vi "Modbus LDO Boolean Decode.vi"(8 "error in":errorcluster, 11 "PLC Data":T1) -> (0 "error out":errorcluster, 3 "PLC Data Out":T1)   [LabVIEW 2020, in "Modbus.lvlib"]
uses:
  Modbus.lvlib
  Modbus PLC Data All.ctl
  Modbus FVIR Control.ctl
  Modbus LDO Control.ctl
  WritingDataFile/Data to Save.ctl
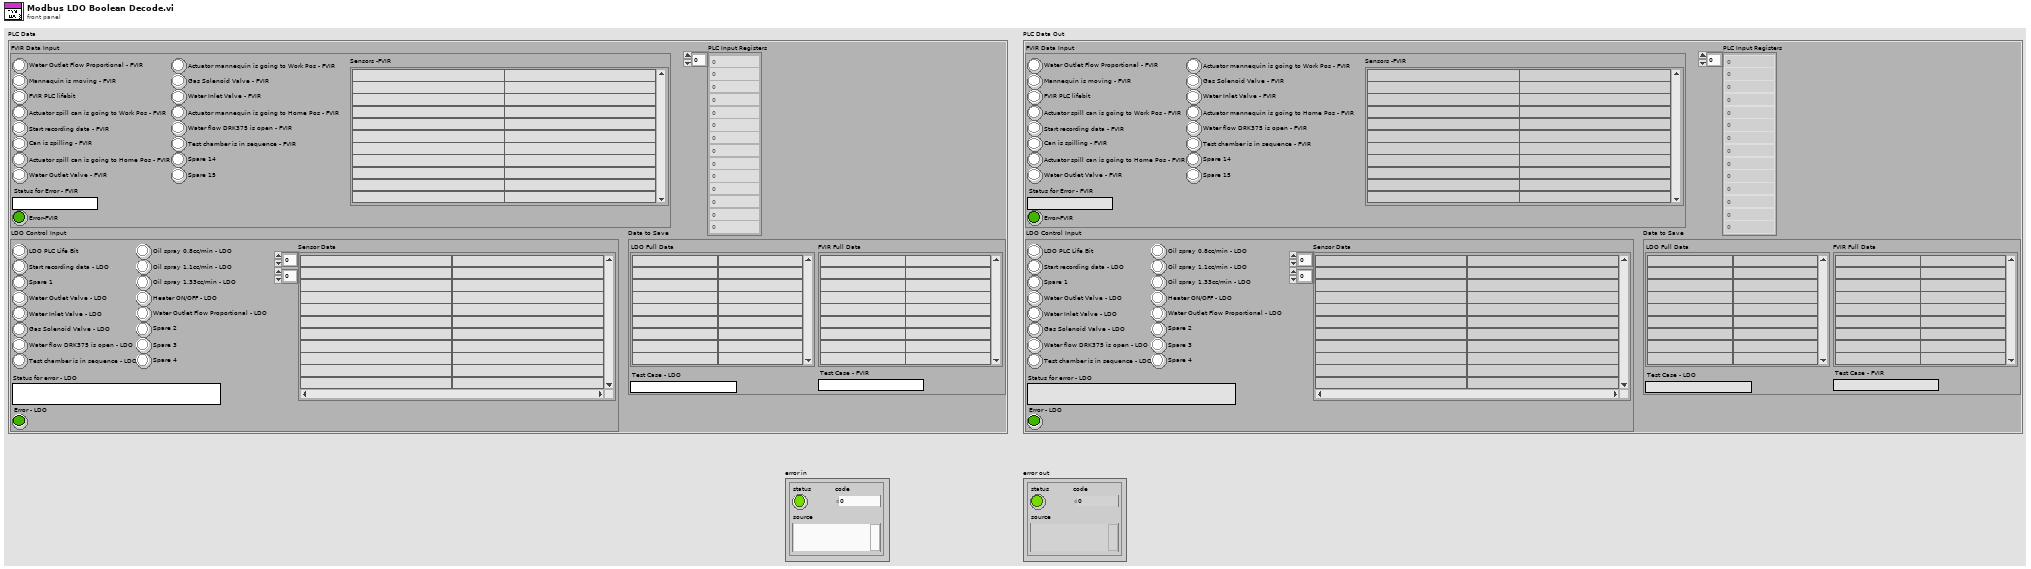
[diagram p1: front panel]
types:
  T1 = typedef "Modbus PLC Data All.ctl" = cluster{"FVIR Data Input":T2, "LDO Control Input":T3, "PLC Input Registers":u16[], "Data to Save":T4}
  T2 = typedef "Modbus FVIR Control.ctl" = cluster{"Spare 15":bool, "Spare 14":bool, "Actuator mannequin is going to Work Pos - FVIR":bool, "Actuator mannequin is going to Home Pos - FVIR":bool, "Test chamber is in sequence - FVIR ":bool, "Water flow DRK375 is open - FVIR":bool, "Gas Solenoid Valve - FVIR":bool, "Water Inlet Valve - FVIR":bool, "Water Outlet Flow Proportional - FVIR":bool, "Start recording data - FVIR":bool, "Actuator spill can is going to Work Pos - FVIR":bool, "Actuator spill can is going to Home Pos - FVIR":bool, "Water Outlet Valve - FVIR":bool, "Can is spilling - FVIR":bool, "Mannequin is moving - FVIR":bool, "FVIR PLC lifebit":bool, "Status for Error - FVIR":string, "Error-FVIR":bool, "Sensors -FVIR":string[][]}
  T3 = typedef "Modbus LDO Control.ctl" = cluster{"LDO PLC Life Bit":bool, "Start recording data - LDO":bool, "Spare 1":bool, "Water Outlet Valve - LDO":bool, "Water Inlet Valve - LDO":bool, "Gas Solenoid Valve - LDO":bool, "Water flow DRK375 is open - LDO":bool, "Test chamber is in sequence - LDO":bool, "Oil spray 0.8cc/min - LDO":bool, "Oil spray 1.1cc/min - LDO":bool, "Oil spray 1.33cc/min - LDO":bool, "Heater ON/OFF - LDO":bool, "Water Outlet Flow Proportional - LDO":bool, "Spare 2":bool, "Spare 3":bool, "Spare 4":bool, "Status for error - LDO":string, "Error - LDO":bool, "Sensor Data":string[][]}
  T4 = typedef "Data to Save.ctl" = cluster{"LDO Full Data":string[][], "FVIR Full Data":string[][], "Test Case - FVIR":string, "Test Case - LDO":string}
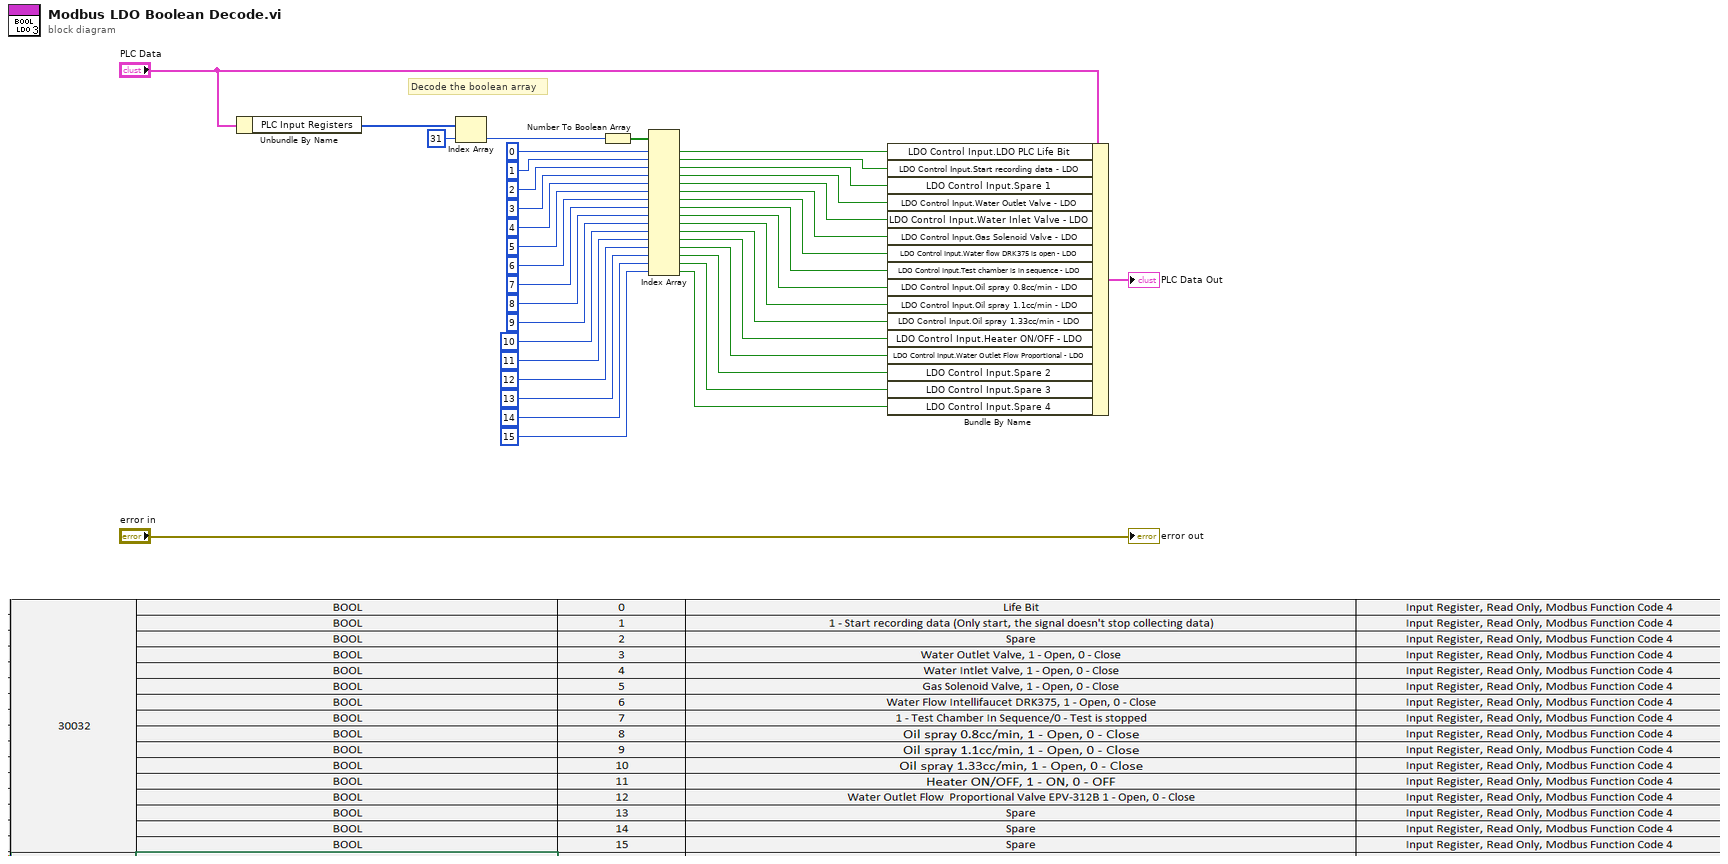
[diagram p0: block diagram]
diagram:
  # "Decode the boolean array"
  n1 = Unbundle By Name("PLC Data") -> ("PLC Input Registers"=w2:u16[])
  n2 = Index Array(array=w2, index=31) -> (element=w39:u16)
  n3 = Number To Boolean Array(number=w39) -> (Boolean array=w38:bool[])
  n4 = Index Array(array=w38, index #1=0 ("index"), index #2=1 ("index"), index #3=2 ("index"), index #4=3 ("index"), index #5=4 ("index"), index #6=5 ("index"), index #7=6 ("index"), index #8=7 ("index"), index #9=8 ("index"), index #10=9 ("index"), index #11=10 ("index"), index #12=11 ("index"), index #13=12 ("index"), index #14=13 ("index"), index #15=14 ("index"), index #16=15 ("index")) -> (element #1=w20:bool, element #2=w19:bool, element #3=w18:bool, element #4=w17:bool, element #5=w16:bool, element #6=w15:bool, element #7=w14:bool, element #8=w13:bool, element #9=w12:bool, element #10=w11:bool, element #11=w10:bool, element #12=w9:bool, element #13=w8:bool, element #14=w7:bool, element #15=w6:bool, element #16=w5:bool)
  n5 = Bundle By Name(cluster="PLC Data", "LDO Control Input.LDO PLC Life Bit"=w20, "LDO Control Input.Start recording data - LDO"=w19, "LDO Control Input.Spare 1"=w18, "LDO Control Input.Water Outlet Valve - LDO"=w17, "LDO Control Input.Water Inlet Valve - LDO"=w16, "LDO Control Input.Gas Solenoid Valve - LDO"=w15, "LDO Control Input.Water flow DRK375 is open - LDO"=w14, "LDO Control Input.Test chamber is in sequence - LDO"=w13, "LDO Control Input.Oil spray 0.8cc/min - LDO"=w12, "LDO Control Input.Oil spray 1.1cc/min - LDO"=w11, "LDO Control Input.Oil spray 1.33cc/min - LDO"=w10, "LDO Control Input.Heater ON/OFF - LDO"=w9, "LDO Control Input.Water Outlet Flow Proportional - LDO"=w8, "LDO Control Input.Spare 2"=w7, "LDO Control Input.Spare 3"=w6, "LDO Control Input.Spare 4"=w5) -> (→"PLC Data Out":T1)
  "error out" <- "error in"
